vi "Architecture Conversion.vi"(0 "Arch In":string) -> (4 "Arch OUT":string)   [LabVIEW 2021, in "Packager Helpers.lvlib"]
uses:
  Packager Helpers.lvlib
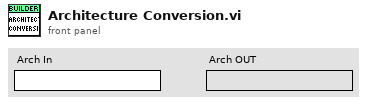
[diagram p1: front panel]
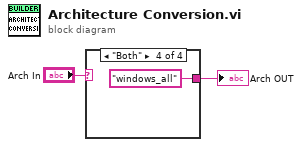
[diagram p0: block diagram]
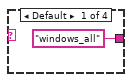
[diagram p2: hidden frame]
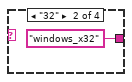
[diagram p3: hidden frame]
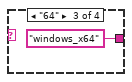
[diagram p4: hidden frame]
diagram:
  n1 = case shown="\"Both\"" "Arch In" {
    tunnel: ["windows_all" ("Arch OUT") "windows_x32" ("Arch OUT") "windows_x64" ("Arch OUT") "windows_all" ("Arch OUT")] -> w1
    frame Default {
    }
    frame "32" {
    }
    frame "64" {
    }
    frame "Both" {
    }
  }
  "Arch OUT" <- w1
